vi "TestPointEditorSts.vi"(6 "TorqueValue":refnum<vi>, 7 "Program_Multi":refnum<vi>, 8 "FetchRate":refnum<vi>, 9 "DwellTime":refnum<vi>, 10 "SpeedValue":refnum<vi>, 11 "index":refnum<vi>) -> ()   [LabVIEW 2024]
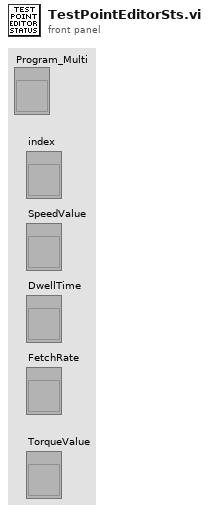
[diagram p1: front panel]
types:
  T1 = enum8{"Enabled", "Disabled", "Disabled and Grayed Out"}
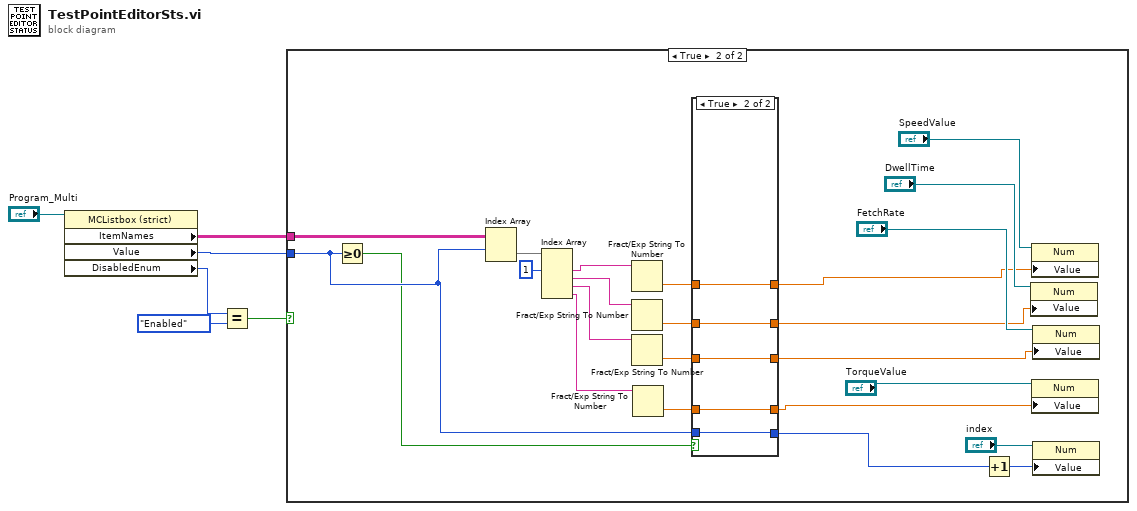
[diagram p0: block diagram]
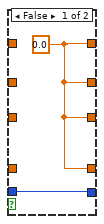
[diagram p3: hidden frame]
diagram:
  n1 = property class="MCListbox (strict)"(reference="Program_Multi") -> ("ItemNames"=w5:string[][], "Value"=w4:i32, "DisabledEnum"=w3:T1)  [unwired: 1 in, 2 out]
  n2 = Equal?(x=w3, y=T1."Enabled") -> (x = y?=w1:bool)
  n3 = case shown="True" w1 {
    tunnel: w5 -> [_ w30]
    tunnel: w4 -> [_ w16]
    frame False {
    }
    frame True {
      n4 = Greater Or Equal To 0?(x=w16) -> (x >= 0?=w15:bool)
      n5 = Index Array(array=w30, index (row)=w16) -> (element=w29:string[])  [unwired: 1 in]
      n6 = Index Array(array=w29, index #1=1 ("index")) -> (element #1=w26:string, element #2=w25:string, element #3=w24:string, element #4=w10:string)  [unwired: 3 in]
      n7 = Fract/Exp String To Number(string=w26) -> (number=w19:dbl)  [unwired: 3 in, 1 out]
      n8 = Fract/Exp String To Number(string=w25) -> (number=w18:dbl)  [unwired: 3 in, 1 out]
      n9 = Fract/Exp String To Number(string=w24) -> (number=w17:dbl)  [unwired: 3 in, 1 out]
      n10 = Fract/Exp String To Number(string=w10) -> (number=w9:dbl)  [unwired: 3 in, 1 out]
      n11 = case shown="True" w15 {
        tunnel: [w31 w37] -> w14
        tunnel: w19 -> [_ w37]
        tunnel: [w31 w36] -> w13
        tunnel: w18 -> [_ w36]
        tunnel: [w31 w35] -> w12
        tunnel: w17 -> [_ w35]
        tunnel: [w32 w34] -> w11
        tunnel: w16 -> [w32 w34]
        tunnel: [w31 w33] -> w7
        tunnel: w9 -> [_ w33]
        frame False {
          w31 = 0.0
        }
        frame True {
        }
      }
      n12 = Increment(x=w11) -> (x+1=w20:i32)
      n13 = property class="Num"(reference="DwellTime", "Value"=w13) -> ()  [unwired: 1 in, 2 out]
      n14 = property class="Num"(reference="SpeedValue", "Value"=w14) -> ()  [unwired: 1 in, 2 out]
      n15 = property class="Num"(reference="TorqueValue", "Value"=w7) -> ()  [unwired: 1 in, 2 out]
      n16 = property class="Num"(reference="FetchRate", "Value"=w12) -> ()  [unwired: 1 in, 2 out]
      n17 = property class="Num"(reference="index", "Value"=w20) -> ()  [unwired: 1 in, 2 out]
    }
  }
